vi "PowerLawFit.vi"(7 "MaxFitZ":dbl, 8 "ZeroDisplacement?":bool, 9 "Zref":dbl, 10 "U/Uref":dbl[](array[numeric]), 11 "z":dbl[](array[numeric])) -> (0 "n":dbl, 1 "PowerLawFitEquation":string, 2 "CroppedData":cluster{"X Out":dbl[], "Y Out":dbl[]}, 3 "FitCurve":T1, 4 "d0":dbl format="%#.2f")   [LabVIEW 2013]
uses:
  <vilib>/Analysis/6fits.llb/Curve Fitting Criteria.ctl
  <vilib>/Analysis/6fits.llb/Remove Outliers (Range).vi
  <vilib>/gmath/NumericalOptimization/Nonlinear Curve Fit LM formula string.vi
  <vilib>/gmath/NI_Gmath.lvlib
  <vilib>/Analysis/NI_AALPro.lvlib
panel:
  in  "d0Estimate":dbl
  in  "nEstimate":dbl=1.0
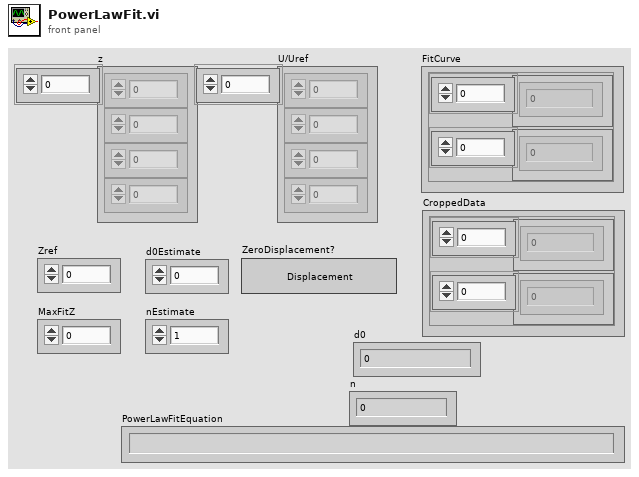
[diagram p1: front panel]
types:
  T1 = cluster{"Array":dbl[], "best nonlinear fit":dbl[]}
  T2 = cluster{"model":string, "Parameters":string[], "x":string}
  T3 = cluster{"amp min":dbl, "amp max":dbl, "power min":dbl, "power max":dbl, "offset min":dbl, "offset max":dbl}
  T4 = typedef "NI_AALPro.lvlib/Curve Fitting Criteria.ctl" = u16
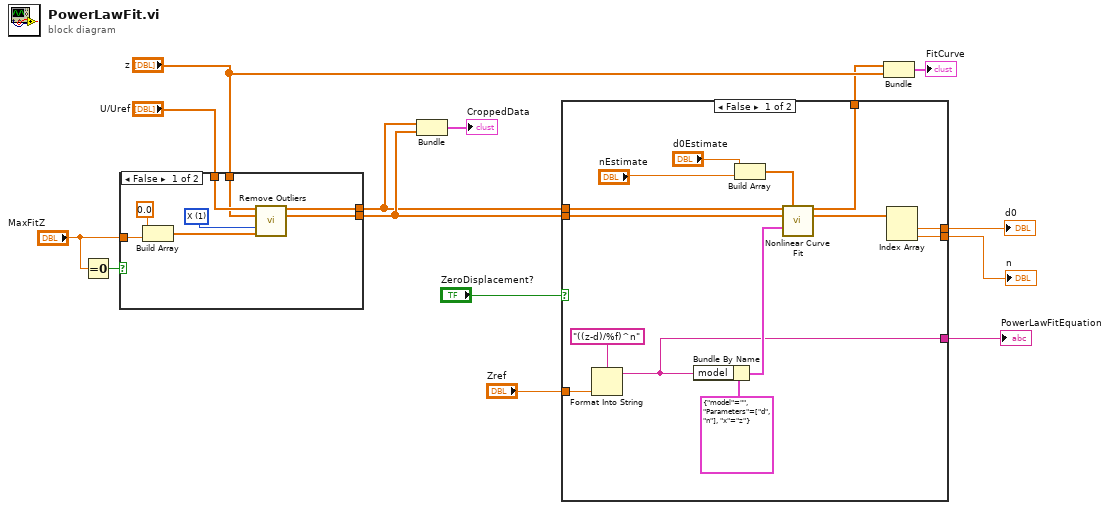
[diagram p0: block diagram]
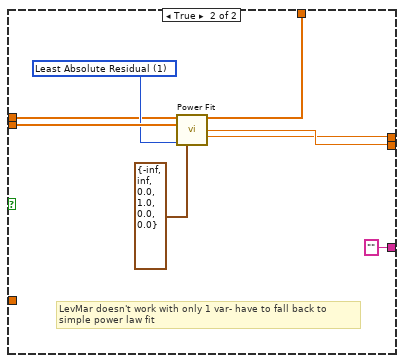
[diagram p2: hidden frame]
diagram:
  n1 = Equal To 0?(x="MaxFitZ") -> (x = 0?=w10:bool)
  n2 = case shown="False" w10 {
    tunnel: [w22 w23] -> w7
    tunnel: [w21 w24] -> w8
    tunnel: "U/Uref" -> [w19 w23]
    tunnel: "z" -> [w17 w24]
    tunnel: "MaxFitZ" -> [w15 _]
    frame False {
      w20 = u16 1 items=["x", "X", "X and Y"] ("range type")
      n3 = Build Array(0.0 ("element"), w15) -> (w16:dbl[])
      n4 = call-poly <vilib>:"Remove Outliers.vi"("Y"=w19, "X"=w17, "range type"=w20, "Range"=w16) -> ("Y Out"=w22:dbl[], "X Out"=w21:dbl[])  [unwired: 7 in, 3 out]
    }
    frame True {
    }
  }
  n5 = Bundle("U/Uref"=w7, "z"=w8) -> (→"CroppedData":cluster{"U/Uref":dbl[], "z":dbl[]})  [unwired: 1 in]
  n6 = case shown="False" "ZeroDisplacement?" {
    tunnel: [w35 ""] -> w9
    tunnel: w8 -> [w34 w41]
    tunnel: w7 -> [w33 w39]
    tunnel: [w32 w43] -> w6
    tunnel: [w31 w45] -> w5
    tunnel: "Zref" -> [w30 _]
    tunnel: [w29 w46] -> w2
    frame False {
      n7 = Format Into String(format string="((z-d)/%f)^n" ("vonKarman Spectrum"), w30) -> (resulting string=w35:string)  [unwired: 2 in, 1 out]
      n8 = Bundle By Name(cluster=T2 {"model"="", "Parameters"=["d", "n"], "x"="z"} ("model description"), "model"=w35) -> (w38:T2)
      n9 = Build Array("d0Estimate", "nEstimate") -> (w36:dbl[])
      n10 = call-poly <vilib>:"Nonlinear Curve Fit.vi"("Y"=w33, "initial parameters"=w36, "X"=w34, "model description"=w38) -> ("best nonlinear fit"=w29:dbl[], "best fit parameters"=w37:dbl[])  [unwired: 7 in, 3 out]
      n11 = Index Array(array=w37) -> (element #1=w32:dbl, element #2=w31:dbl)  [unwired: 2 in]
    }
    frame True {
      w40 = T4 1 items=["Least Square", "Least Absolute Residual", "Bisquare"] ("method")
      # "LevMar doesn't work with only 1 var- have to fall back to\nsimple power law fit"
      n12 = call <vilib>:"Power Fit.vi"("Y"=w39, "X"=w41, "method"=w40, "parameter bounds"=T3 {"amp min"=-inf, "amp max"=inf, "power min"=0.0, "power max"=1.0, "offset min"=0.0, "offset max"=0.0}) -> ("Best Power Fit"=w46:dbl[], "power"=w45:dbl, "offset"=w43:dbl)  [unwired: 6 in, 3 out]
    }
  }
  "n" <- w5
  "PowerLawFitEquation" <- w9
  "d0" <- w6
  n13 = Bundle("Best Power Fit"=w2, "z"="z") -> (→"FitCurve":cluster{"Best Power Fit":dbl[], "z":dbl[]})  [unwired: 1 in]
